vi "Get Scores from XML.vi"(11 "XML In":string) -> (3 "Team_Scores_And_Rankings_Array":T2(array[cluster]))   [LabVIEW 2013]
uses:
  Round_And_Score_Ctrl.ctl
  <vilib>/xml/Close Reference(Node).vi
  <vilib>/xml/NI_XML.lvlib
  <resource>/objmgr/DOMUserDefRef.rc
panel:
  out "error out":errorcluster
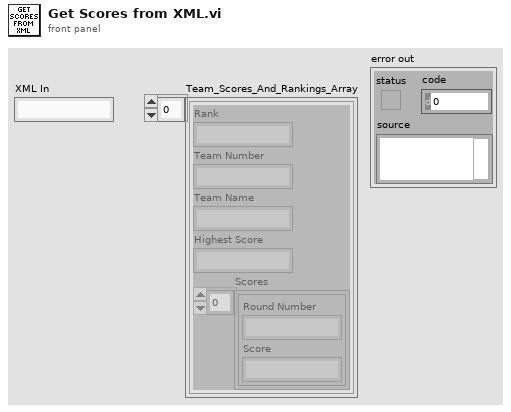
[diagram p1: front panel]
types:
  T1 = typedef "Round_And_Score_Ctrl.ctl" = cluster{"Score":string, "Round Number":string}
  T2 = cluster{"Rank":string, "Team Number":string, "Team Name":string, "Highest Score":string, "Scores":T1[]}[]
  T3 = cluster{"Rank":string, "Team Number":string, "Team Name":string, "Highest Score":string, "Scores":T1[]}
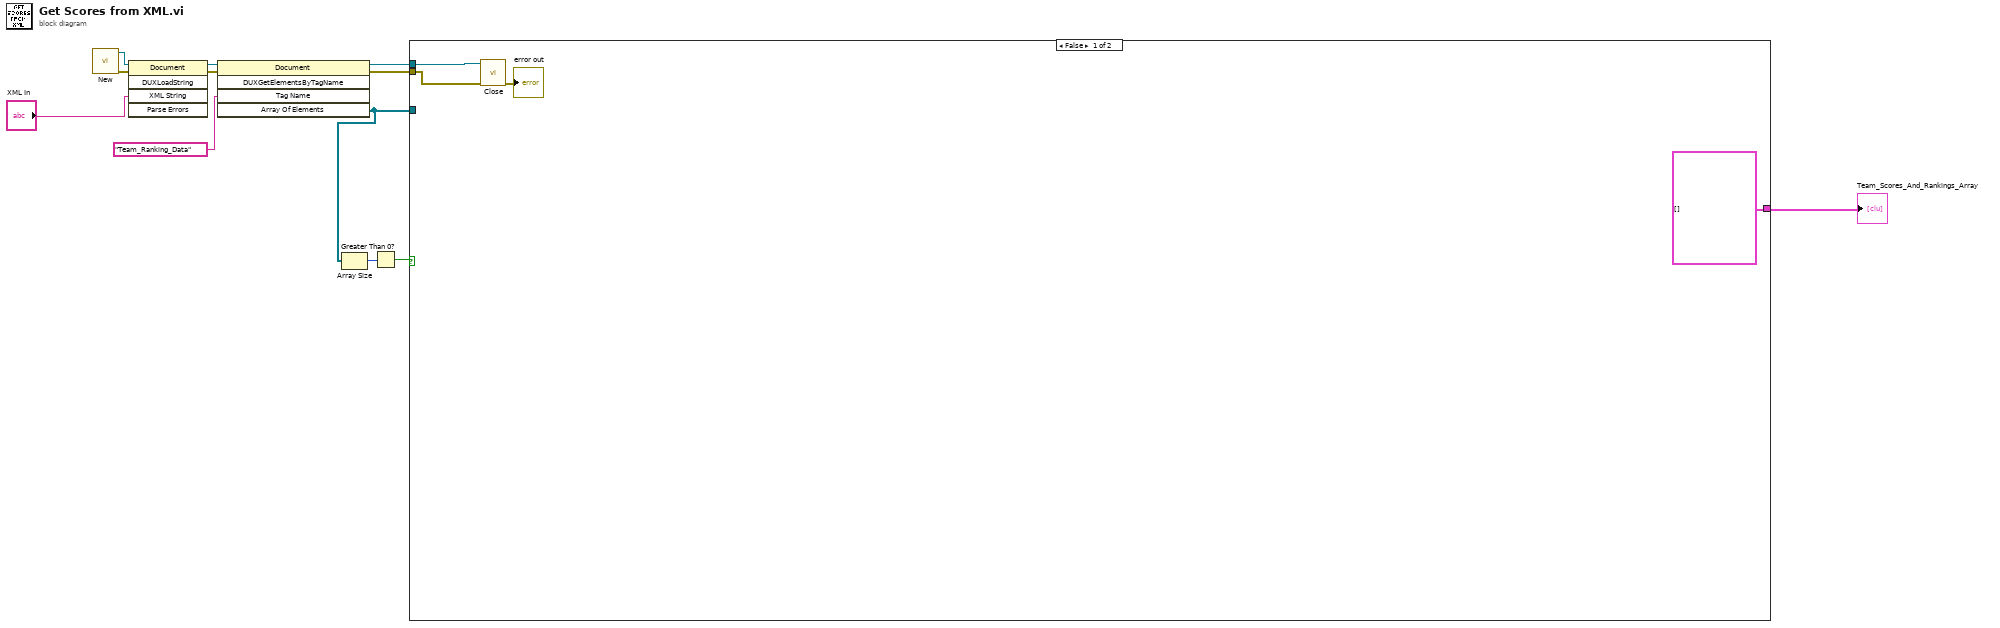
[diagram p0: block diagram]
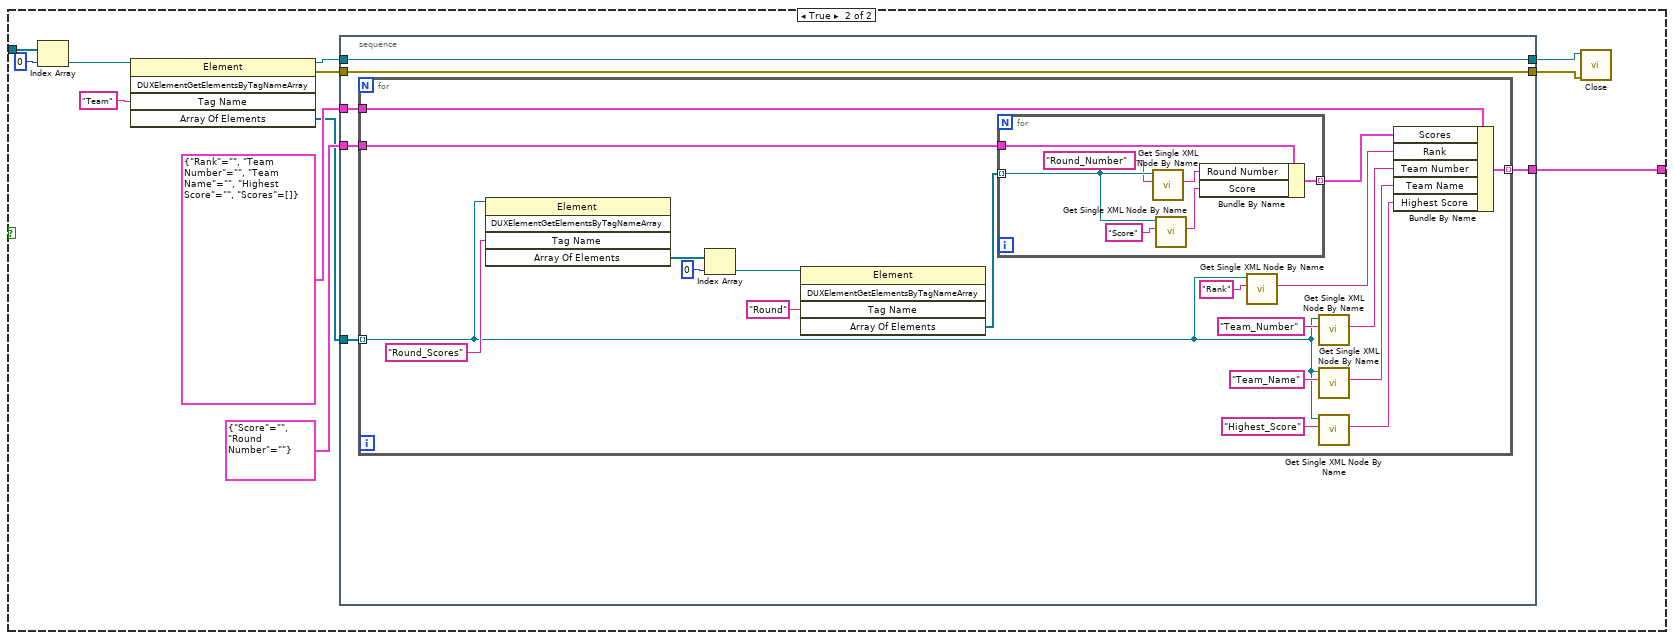
[diagram p2: hidden frame]
diagram:
  n1 = call <vilib>:"New.vi"() -> ("error out"=w6:errorcluster, "DOM document out"=w9:refnum<k20>)  [unwired: 8 in]
  n2 = invoke class="Document" method="DUXLoadString"(reference=w9, error in=w6, "XML String"="XML In") -> (reference out=w8:refnum<k20>, error out=w7:errorcluster)  [unwired: 2 in, 3 out]
  n3 = invoke class="Document" method="DUXGetElementsByTagName"(reference=w8, error in=w7, "Tag Name"="Team_Ranking_Data") -> (reference out=w5:refnum<k20>, error out=w4:errorcluster, "Array Of Elements"=w1:refnum<k20>[])  [unwired: 2 in, 2 out]
  n4 = Array Size(array=w1) -> (size(s)=w3:i32)
  n5 = Greater Than 0?(x=w3) -> (x > 0?=w2:bool)
  n6 = case shown="False" w2 {
    tunnel: [T2 [] w28] -> w12
    tunnel: w1 -> [_ w22]
    tunnel: w4 -> [w15 _]
    tunnel: w5 -> [w16 _]
    frame False {
      n7 = call-poly <vilib>:"Close.vi"("error in (no error)"=w15, "node"=w16) -> ("error out"=→"error out":errorcluster)  [unwired: 7 in]
    }
    frame True {
      n8 = Index Array(array=w22, index=0) -> (element=w17:refnum<k20>)
      n9 = invoke class="Element" method="DUXElementGetElementsByTagNameArray"(reference=w17, "Tag Name"="Team") -> (reference out=w21:refnum<k20>, error out=w20:errorcluster, "Array Of Elements"=w25:refnum<k20>[])  [unwired: 3 in, 2 out]
      n10 = stacked-sequence {
        tunnel: [w34] -> w28
        tunnel: T3 {"Rank"="", "Team Number"="", "Team Name"="", "Highest Score"="", "Scores"=[]} -> [w33]
        tunnel: T1 {"Score"="", "Round Number"=""} -> [w32]
        tunnel: w25 -> [w31]
        tunnel: w21 -> [w30]
        tunnel: [w30] -> w19
        tunnel: w20 -> [w29]
        tunnel: [w29] -> w18
        frame #0 {
          n11 = for {
            tunnel: w31 -> [w48] mode=indexing
            tunnel: w32 -> [w47]
            tunnel: w33 -> [w41]
            tunnel: [w35] -> w34 mode=indexing
            n12 = invoke class="Element" method="DUXElementGetElementsByTagNameArray"(reference=w48, "Tag Name"="Round_Scores") -> ("Array Of Elements"=w43:refnum<k20>[])  [unwired: 3 in, 4 out]
            n13 = Index Array(array=w43, index=0) -> (element=w42:refnum<k20>)
            n14 = invoke class="Element" method="DUXElementGetElementsByTagNameArray"(reference=w42, "Tag Name"="Round") -> ("Array Of Elements"=w45:refnum<k20>[])  [unwired: 3 in, 4 out]
            n15 = for {
              tunnel: w45 -> [w60] mode=indexing
              tunnel: w47 -> [w57]
              tunnel: [w54] -> w40 mode=indexing
              n16 = call "Get Single XML Node By Name.vi"("Tag Name"="Round_Number", "Parent Element"=w60) -> ("node text"=w55:string)  [unwired: 7 in, 2 out]
              n17 = call "Get Single XML Node By Name.vi"("Tag Name"="Score", "Parent Element"=w60) -> ("node text"=w56:string)  [unwired: 7 in, 2 out]
              n18 = Bundle By Name(cluster=w57, "Round Number"=w55, "Score"=w56) -> (w54:T1)
            }
            n19 = call "Get Single XML Node By Name.vi"("Tag Name"="Rank", "Parent Element"=w48) -> ("node text"=w39:string)  [unwired: 7 in, 2 out]
            n20 = call "Get Single XML Node By Name.vi"("Tag Name"="Team_Number", "Parent Element"=w48) -> ("node text"=w38:string)  [unwired: 7 in, 2 out]
            n21 = call "Get Single XML Node By Name.vi"("Tag Name"="Team_Name", "Parent Element"=w48) -> ("node text"=w37:string)  [unwired: 7 in, 2 out]
            n22 = call "Get Single XML Node By Name.vi"("Tag Name"="Highest_Score", "Parent Element"=w48) -> ("node text"=w36:string)  [unwired: 7 in, 2 out]
            n23 = Bundle By Name(cluster=w41, "Scores"=w40, "Rank"=w39, "Team Number"=w38, "Team Name"=w37, "Highest Score"=w36) -> (w35:T3)
          }
        }
      }
      n24 = call-poly <vilib>:"Close.vi"("error in (no error)"=w18, "node"=w19) -> ()  [unwired: 7 in, 1 out]
    }
  }
  "Team_Scores_And_Rankings_Array" <- w12
